vi "DataVIS_Select_Intensity_Array.vi"(8 "error in (no error)":errorcluster, 10 "dI/dV 2T 2":cluster{dbl[], dbl[]}[][][](array[cluster]), 11 "State Wire IN":T1) -> (0 "error out":errorcluster, 2 "Intensity Array OUT":cluster{dbl[], dbl[]}[](array[cluster]), 3 "State Wire OUT":T1)   [LabVIEW 2016]
uses:
  DataVIS_StateWire.ctl
  <vilib>/Utility/miscctls.llb/LVPointDoubleTypeDef.ctl
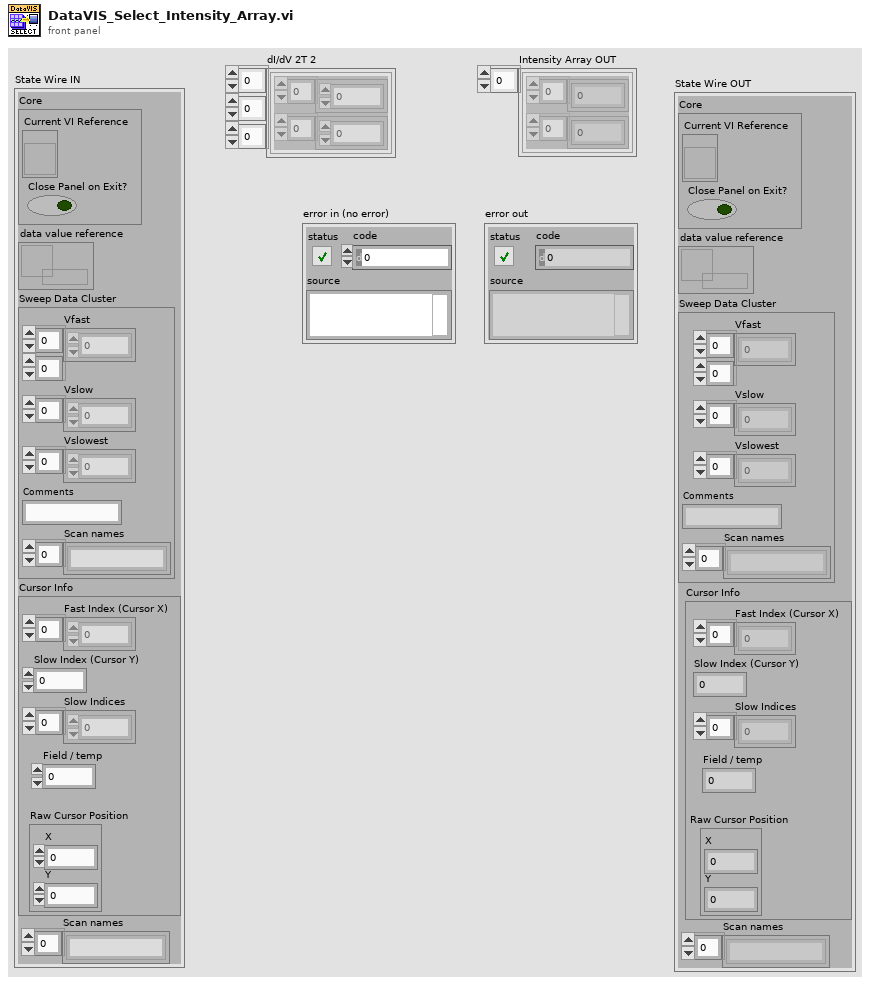
[diagram p1: front panel]
types:
  T1 = typedef "DataVIS_StateWire.ctl" = cluster{"Core":cluster{"Current VI Reference":refnum<vi>, "Close Panel on Exit?":bool}, "data value reference":refnum<data-value>, "Sweep Data Cluster":cluster{"Vfast":dbl[][], "Vslow":dbl[], "Vslowest":dbl[], "Comments":string, "Scan names":string[]}, "Cursor Info":cluster{"Fast Index (Cursor X)":dbl[], "Slow Index (Cursor Y)":dbl, "Slow Indices":dbl[], "Raw Cursor Position":T2, "Field / temp":i32}, "Scan names":string[]}
  T2 = typedef "LVPointDoubleTypeDef.ctl" = cluster{"X":dbl, "Y":dbl}
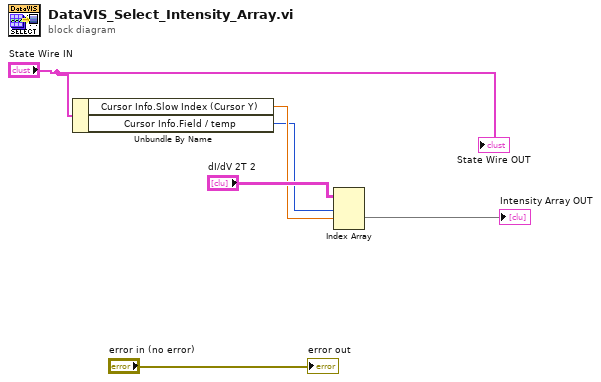
[diagram p0: block diagram]
diagram:
  n1 = Unbundle By Name("State Wire IN") -> ("Cursor Info.Slow Index (Cursor Y)"=w4:dbl, "Cursor Info.Field / temp"=w2:i32)
  n2 = Index Array(array="dI/dV 2T 2", index (dim 0)=w2, index (dim 1)=w4) -> (element=→"Intensity Array OUT":cluster{dbl[], dbl[]}[])  [unwired: 1 in]
  "error out" <- "error in (no error)"
  "State Wire OUT" <- "State Wire IN"
